vi "testVisaResource_VXI GPIB-VXI MBD Instr.vi"(8 "error in (no error)":errorcluster, 11 "TestCase in":refnum<class "EasyXMLTest.lvclass">) -> (0 "error out":errorcluster, 3 "TestCase out":refnum<class "EasyXMLTest.lvclass">)   [LabVIEW 2011, in "EasyXMLTest.lvclass"]
doc: "Verify that error in is not overwritten"
uses:
  EasyXMLTest.lvclass
panel:
  out "Produced Data":variant
  out "Input Data":variant
  out "XML String":string
  out "Generated XML String":string
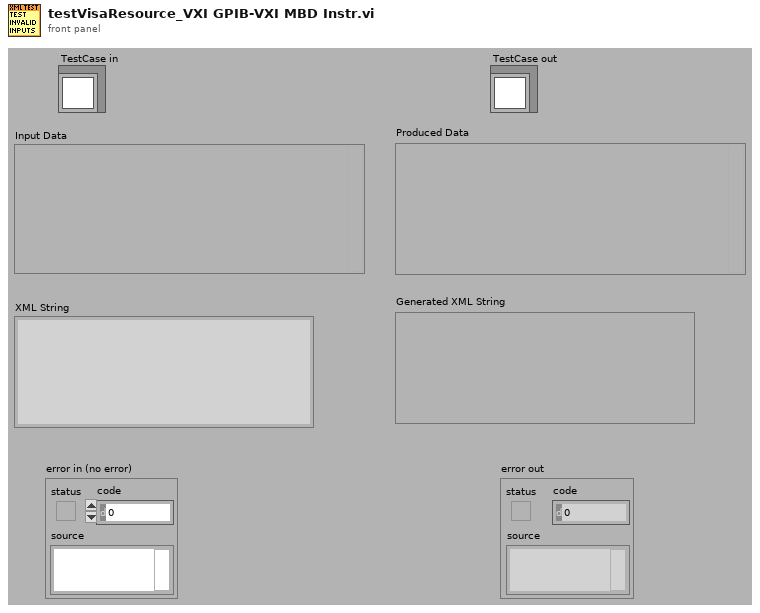
[diagram p1: front panel]
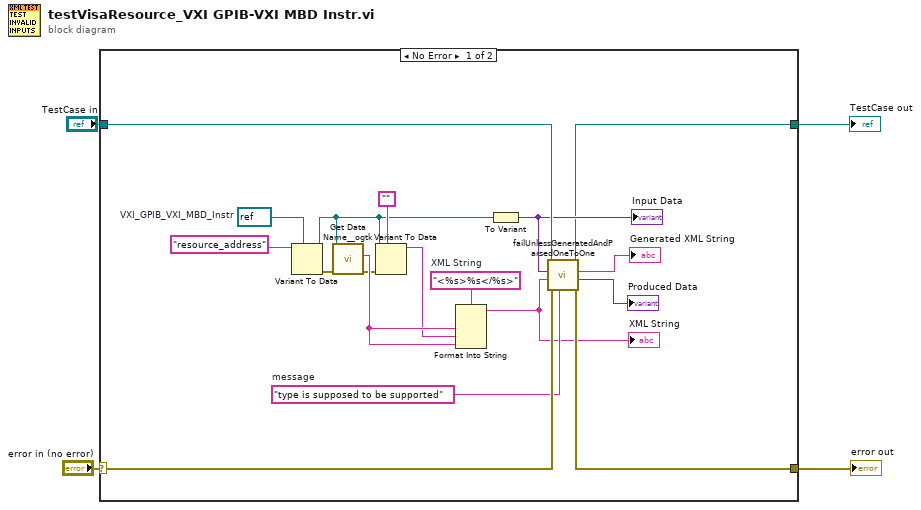
[diagram p0: block diagram]
diagram:
  n1 = case shown="No Error" "error in (no error)" {
    selector: "error in (no error)" -> [w21 w24]
    tunnel: [w16 w24] -> w2
    tunnel: [w15 w23] -> w1
    tunnel: "TestCase in" -> [w22 w23]
    frame No Error {
      w5 = refnum<visa-resource-name> refnum  # VXI_GPIB_VXI_MBD_Instr
      w12 = "<%s>%s</%s>"  # XML String
      w20 = "type is supposed to be supported"  # message
      n2 = Variant To Data(type=w5, Variant="resource_address") -> (data=w6:refnum<visa-resource-name>, error out=w8:errorcluster)  [unwired: 1 in]
      n3 = call <userlib>:"Get Data Name__ogtk.vi"("error in (no error)"=w8, "Data"=w6) -> ("error out"=w9:errorcluster, "Data Name"=w13:string)  [unwired: 7 in, 1 out]
      n4 = Variant To Data(error in=w9, type="", Variant=w6) -> (data=w10:string)  [unwired: 1 out]
      n5 = Format Into String(format string=w12, w13, w10, w13) -> (resulting string=w11:string)  [unwired: 2 in, 1 out]
      "XML String" <- w11
      n6 = To Variant(anything=w6) -> (Variant=w18:variant)
      "Input Data" <- w18
      n7 = call "failUnlessGeneratedAndParsedOneToOne.vi"("message (\"\")"=w20, "error in"=w21, "XML String"=w11, "Data"=w18, "EasyXMLTest in"=w22) -> ("error out"=w16:errorcluster, "Produced Data"=→"Produced Data":variant, "Generated XML String"=→"Generated XML String":string, "EasyXMLTest out"=w15:refnum<class "EasyXMLTest.lvclass">)  [unwired: 3 in]
    }
    frame Error {
    }
  }
  "error out" <- w2
  "TestCase out" <- w1
